vi "caculatekinematics.vi"(2 "Input attitude array":dbl[](array[numeric])) -> (0 "output PWM":T2, 1 "length of each link":T1)   [LabVIEW 2018]
uses:
  <vilib>/Analysis/baseanly.llb/Real A x B.vi
  <vilib>/Analysis/_algsub.llb/Real Vector Norm.vi
  <vilib>/Analysis/Matrix/Numeric/Subtract/Subtract - RM,RM.vi
  <vilib>/Analysis/Matrix/Numeric/Add/Add - RM,RM.vi
  <vilib>/Analysis/NI_AALBase.lvlib
  <vilib>/Analysis/NI_AALPro.lvlib
  <vilib>/Analysis/Matrix/NI_Matrix.lvlib
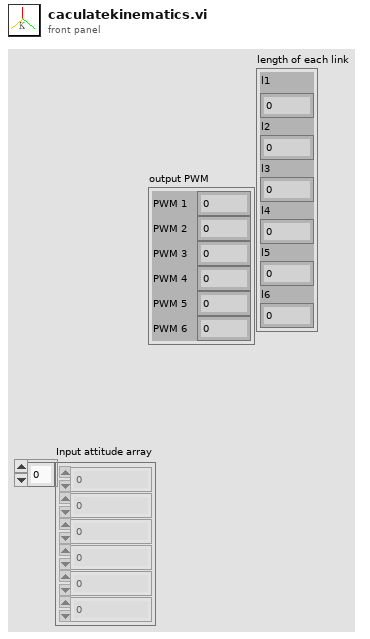
[diagram p1: front panel]
types:
  T1 = cluster{"l1":dbl, "l2":dbl, "l3":dbl, "l4":dbl, "l5":dbl, "l6":dbl}
  T2 = cluster{"PWM 1":dbl, "PWM 2":dbl, "PWM 3":dbl, "PWM 4":dbl, "PWM 5":dbl, "PWM 6":dbl}
  T3 = typedef "NI_Matrix.lvlib/RealMatrix.ctl" = dbl[][]
  T4 = cluster{"norm":dbl, "norm":dbl, "norm":dbl, "norm":dbl, "norm":dbl, "norm":dbl}
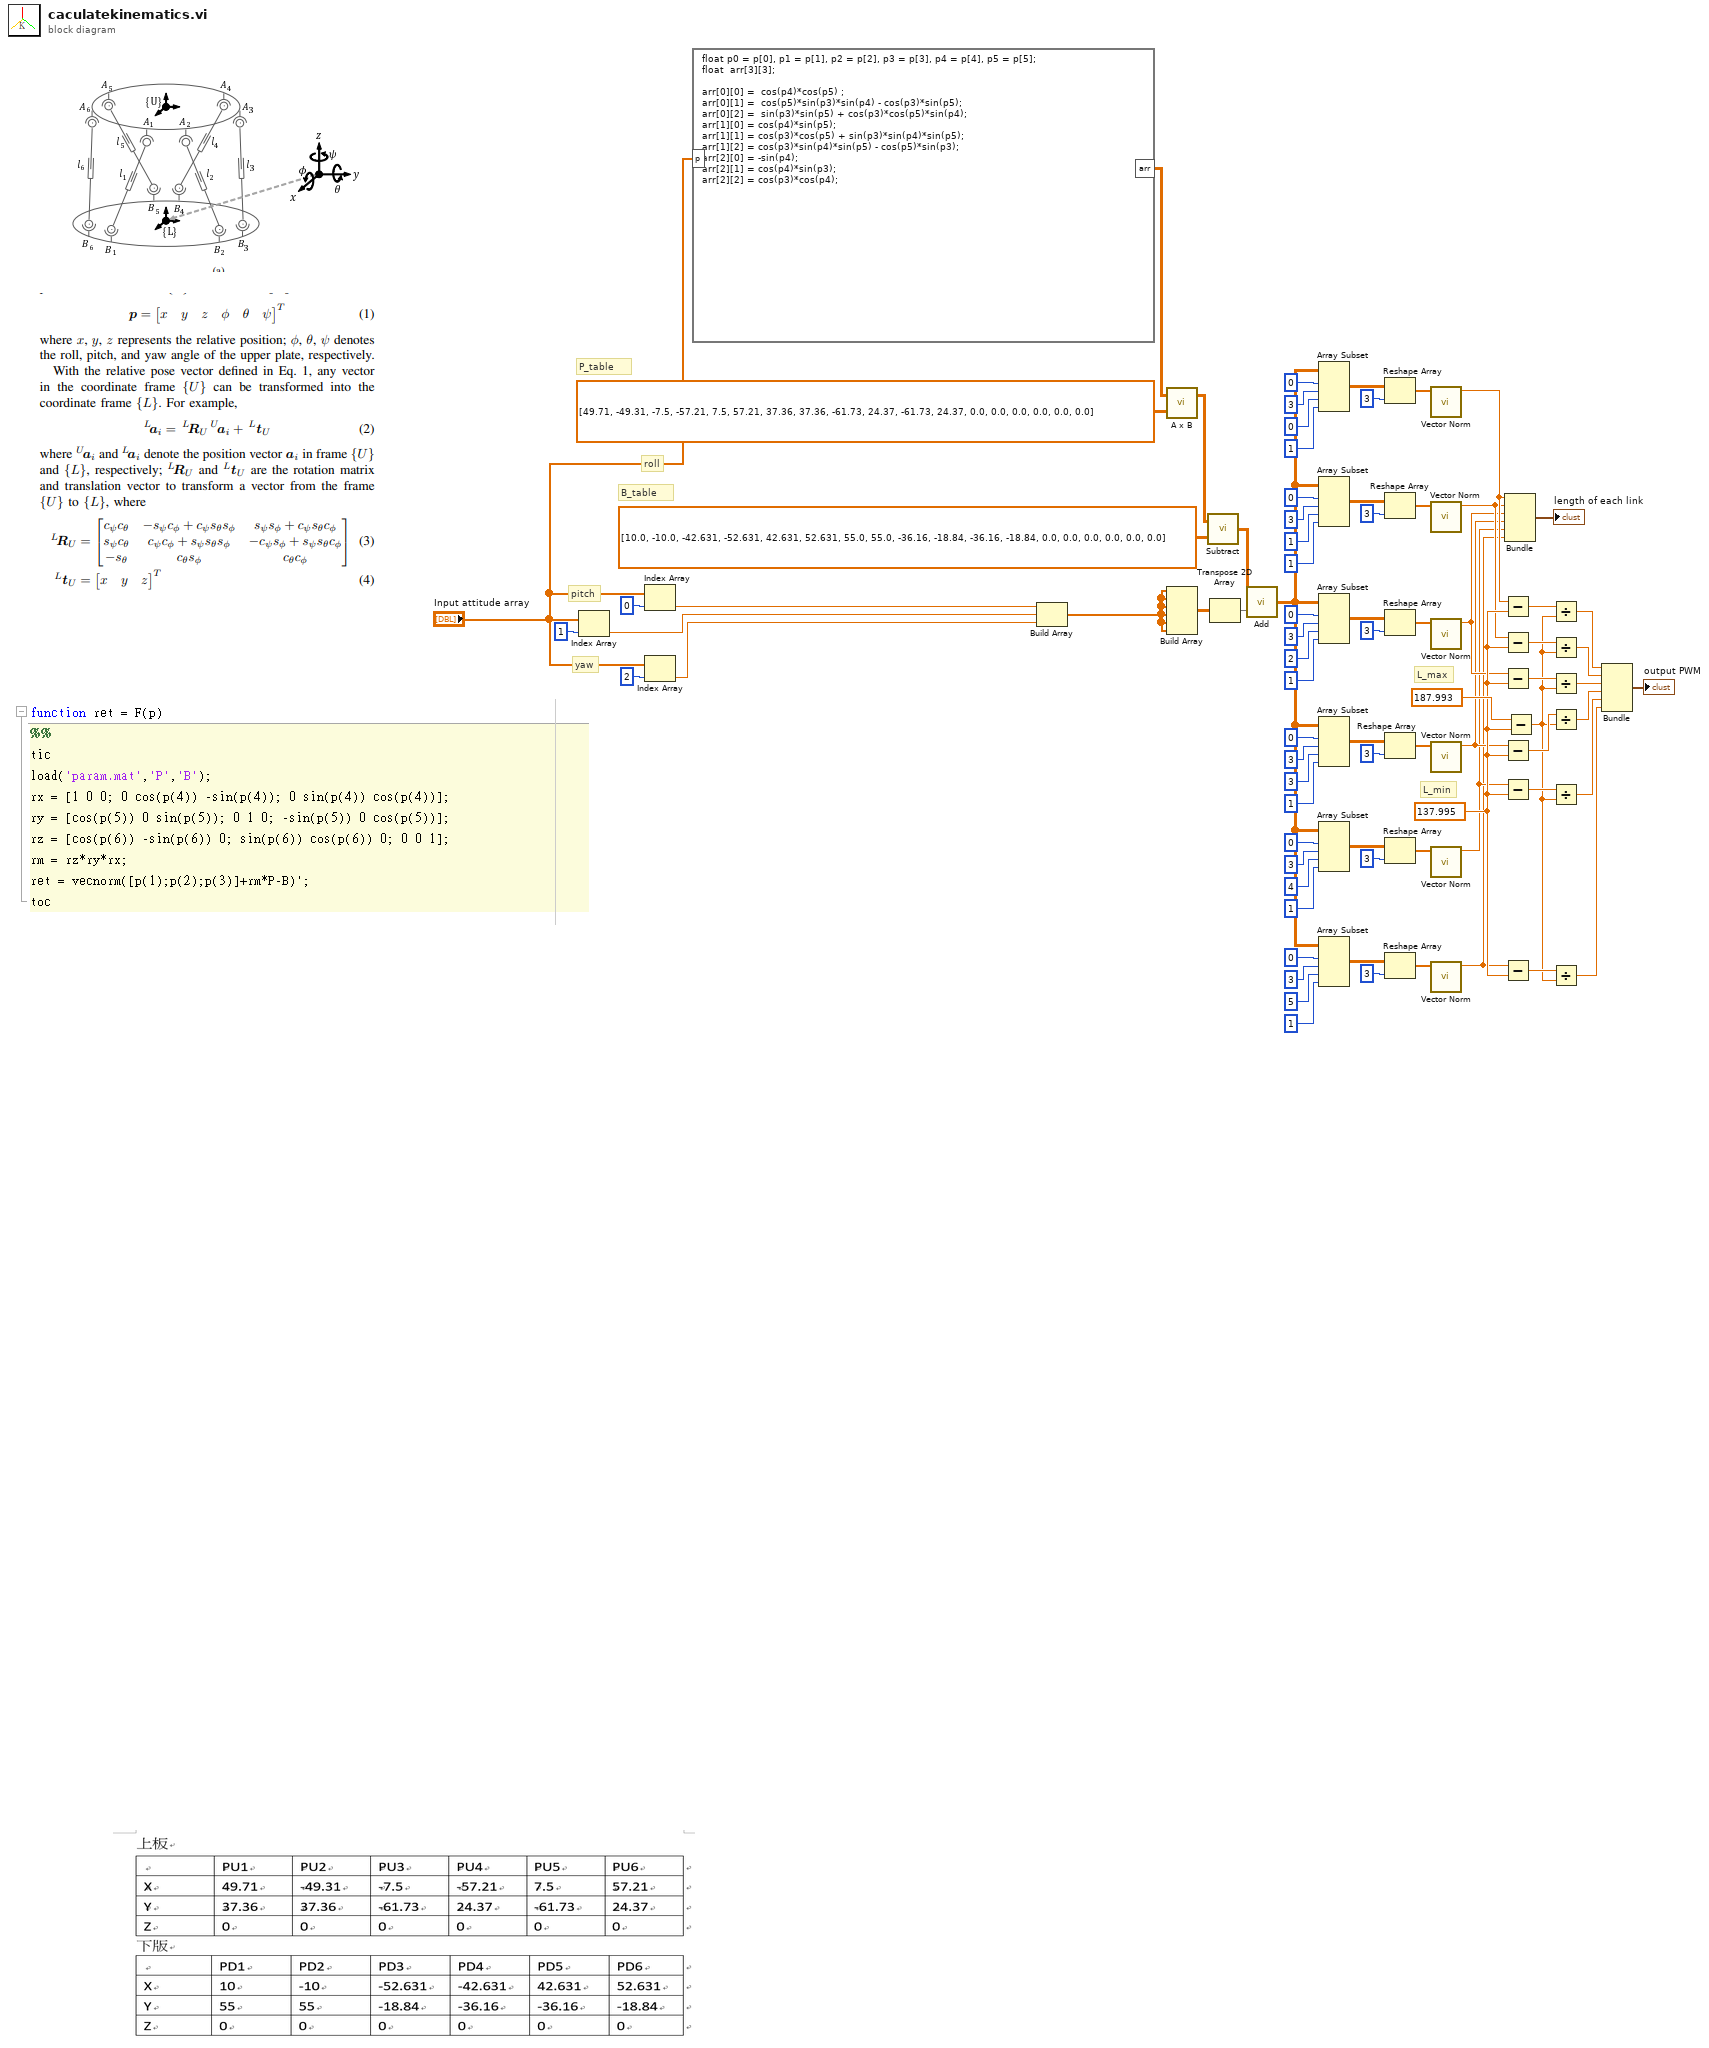
[diagram p0: block diagram]
diagram:
  w15 = 137.995
  # "yaw"
  # "pitch"
  # "roll"
  # "P_table"
  # "B_table"
  # "L_min"
  # "L_max"
  n1 = Index Array(array="Input attitude array", index=1) -> (element=w76:dbl)
  n2 = Index Array(array="Input attitude array", index=0) -> (element=w77:dbl)
  n3 = Index Array(array="Input attitude array", index=2) -> (element=w75:dbl)
  n4 = formula code="float p0 = p[0], p1 = p[1], p2 = p[2], p3 = p[3], p4 = p[4], p5 = p[5];\nfloat  arr[3][3];\n\narr[0][0] =  cos(p4)*cos(p5) ;\narr[0][1] =  cos(p5)*sin(p3)*sin(p4) - cos(p3)*sin(p5);\narr[0][2] =  sin(p3)*sin(p5) + cos(p3)*cos(p5)*sin(p4);\narr[1][0] = cos(p4)*sin(p5);\narr[1][1] = cos(p3)*cos(p5) + sin(p3)*sin(p4)*sin(p5);\narr[1][2] = cos(p3)*sin(p4)*sin(p5) - cos(p5)*sin(p3);\narr[2][0] = -sin(p4);\narr[2][1] = cos(p4)*sin(p3);\narr[2][2] = cos(p3)*cos(p4);"("p"="Input attitude array") -> ("arr"=w32:dbl[][])
  n5 = Build Array(w77, w76, w75) -> (w26:dbl[])
  n6 = call-poly <vilib>:"A x B.vi"("B"=dbl[][] [[49.71, -49.31, -7.5, -57.21, 7.5, 57.21], [37.36, 37.36, -61.73, 24.37, -61.73, 24.37], [0.0, 0.0, 0.0, 0.0, 0.0, 0.0]], "A"=w32) -> ("A x B"=w30:T3)  [unwired: 1 out]
  n7 = Build Array(w26, w26, w26, w26, w26, w26) -> (w25:dbl[][])
  n8 = call-poly <vilib>:"Subtract.vi"("Real Matrix B"=dbl[][] [[10.0, -10.0, -42.631, -52.631, 42.631, 52.631], [55.0, 55.0, -36.16, -18.84, -36.16, -18.84], [0.0, 0.0, 0.0, 0.0, 0.0, 0.0]], "Real Matrix A"=w30) -> ("A - B"=w29:T3)
  n9 = Transpose 2D Array(2D array=w25) -> (transposed array=w24:dbl[][])
  n10 = call-poly <vilib>:"Add.vi"("Real Matrix B"=w24, "Real Matrix A"=w29) -> ("A + B"=w28:T3)
  n11 = Array Subset(array=w28, index (row)=0 ("index"), length (row)=3 ("length"), index (col)=0 ("index"), length (col)=1 ("length")) -> (w50:T3)
  n12 = Array Subset(array=w28, index (row)=0 ("index"), length (row)=3 ("length"), index (col)=1 ("index"), length (col)=1 ("length")) -> (w45:T3)
  n13 = Array Subset(array=w28, index (row)=0 ("index"), length (row)=3 ("length"), index (col)=2 ("index"), length (col)=1 ("length")) -> (w42:T3)
  n14 = Array Subset(array=w28, index (row)=0 ("index"), length (row)=3 ("length"), index (col)=3 ("index"), length (col)=1 ("length")) -> (w39:T3)
  n15 = Array Subset(array=w28, index (row)=0 ("index"), length (row)=3 ("length"), index (col)=4 ("index"), length (col)=1 ("length")) -> (w36:T3)
  n16 = Array Subset(array=w28, index (row)=0 ("index"), length (row)=3 ("length"), index (col)=5 ("index"), length (col)=1 ("length")) -> (w33:T3)
  n17 = Reshape Array(w50, 3 ("dimension size")) -> (w48:dbl[])
  n18 = Reshape Array(w45, 3 ("dimension size")) -> (w46:dbl[])
  n19 = Reshape Array(w42, 3 ("dimension size")) -> (w43:dbl[])
  n20 = Reshape Array(w39, 3 ("dimension size")) -> (w40:dbl[])
  n21 = Reshape Array(w36, 3 ("dimension size")) -> (w37:dbl[])
  n22 = Reshape Array(w33, 3 ("dimension size")) -> (w34:dbl[])
  n23 = call-poly <vilib>:"Vector Norm.vi"("Input Vector"=w48) -> ("norm"=w7:dbl)  [unwired: 9 in, 1 out]
  n24 = call-poly <vilib>:"Vector Norm.vi"("Input Vector"=w46) -> ("norm"=w6:dbl)  [unwired: 9 in, 1 out]
  n25 = call-poly <vilib>:"Vector Norm.vi"("Input Vector"=w43) -> ("norm"=w5:dbl)  [unwired: 9 in, 1 out]
  n26 = call-poly <vilib>:"Vector Norm.vi"("Input Vector"=w40) -> ("norm"=w4:dbl)  [unwired: 9 in, 1 out]
  n27 = call-poly <vilib>:"Vector Norm.vi"("Input Vector"=w37) -> ("norm"=w3:dbl)  [unwired: 9 in, 1 out]
  n28 = call-poly <vilib>:"Vector Norm.vi"("Input Vector"=w34) -> ("norm"=w2:dbl)  [unwired: 9 in, 1 out]
  n29 = Subtract(x=w7, y=w15) -> (x-y=w17:dbl)
  n30 = Subtract(x=w6, y=w15) -> (x-y=w18:dbl)
  n31 = Subtract(x=w5, y=w15) -> (x-y=w19:dbl)
  n32 = Subtract(x=w4, y=w15) -> (x-y=w20:dbl)
  n33 = Subtract(x=w3, y=w15) -> (x-y=w21:dbl)
  n34 = Subtract(x=w2, y=w15) -> (x-y=w22:dbl)
  n35 = Bundle("norm"=w7, "norm"=w6, "norm"=w5, "norm"=w4, "norm"=w3, "norm"=w2) -> (→"length of each link":T4)  [unwired: 1 in]
  n36 = Subtract(x=187.993, y=w15) -> (x-y=w16:dbl)
  n37 = Divide(x=w17, y=w16) -> (x/y=w14:dbl)
  n38 = Divide(x=w18, y=w16) -> (x/y=w13:dbl)
  n39 = Divide(x=w19, y=w16) -> (x/y=w12:dbl)
  n40 = Divide(x=w20, y=w16) -> (x/y=w11:dbl)
  n41 = Divide(x=w21, y=w16) -> (x/y=w10:dbl)
  n42 = Divide(x=w22, y=w16) -> (x/y=w9:dbl)
  n43 = Bundle(w14, w13, w12, w11, w10, w9) -> (→"output PWM":cluster{dbl, dbl, dbl, dbl, dbl, dbl})  [unwired: 1 in]
